vi "MS SQL_Read_STN_Count.vi"(8 "error in (no error)":errorcluster, 9 "Table?":string, 10 "Query":string, 11 "Refnum in":T1) -> (0 "error out":errorcluster, 1 "RFID":string[](array[string]), 2 "Count":i64, 3 "Refnum out":T1)   [LabVIEW 2020]
uses:
  <vilib>/addons/database/Connection.llb/Conn ObjectReference.ctl
  <vilib>/addons/database/NI_Database_API.lvlib
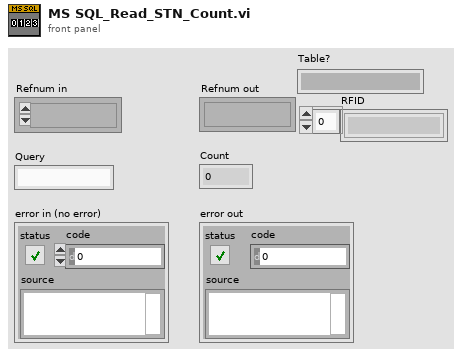
[diagram p1: front panel]
types:
  T1 = typedef "NI_Database_API.lvlib/Conn ObjectReference.ctl" = refnum<k1>
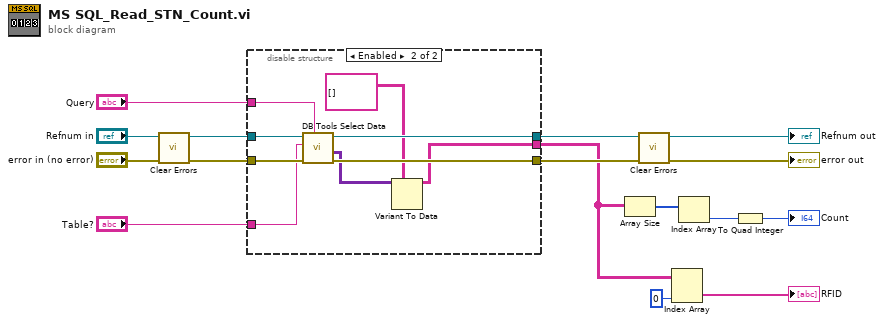
[diagram p0: block diagram]
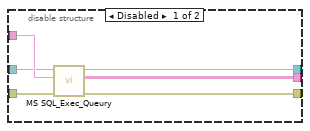
[diagram p2: hidden frame]
diagram:
  n1 = call <vilib>:"Clear Errors.vi"("error in (no error)"="error in (no error)") -> ("error out"=w1:errorcluster)  [unwired: 5 in, 1 out]
  n2 = disable-structure shown="Enabled" {
    disable-tunnel: [w20 w22] -> w4
    disable-tunnel: "Query" -> [w19 w28]
    disable-tunnel: "Refnum in" -> [w18 w29]
    disable-tunnel: w1 -> [w17 w27]
    disable-tunnel: [w16 w26] -> w11
    disable-tunnel: [w15 w25] -> w10
    disable-tunnel: "Table?" -> [_ w21]
    frame Disabled {
      n3 = call "MS SQL_Exec_Queury.vi"("error in (no error)"=w17, "Query"=w19, "Refnum in"=w18) -> ("error out"=w15:errorcluster, "Data"=w20:string[][], "Refnum out"=w16:T1)  [unwired: 5 in, 1 out]
    }
    frame Enabled {
      n4 = call <vilib>:"DB Tools Select Data.vi"("condition"=w28, "error in (no error)"=w27, "table"=w21, "connection reference"=w29) -> ("error out"=w25:errorcluster, "data"=w24:variant[][], "connection reference out"=w26:T1)  [unwired: 2 in]
      n5 = Variant To Data(type=string[][] [] ("Data"), Variant=w24) -> (data=w22:string[][])  [unwired: 1 in, 1 out]
    }
  }
  "Refnum out" <- w11
  n6 = Array Size(array=w4) -> (size(s)=w8:i32[])
  n7 = call <vilib>:"Clear Errors.vi"("error in (no error)"=w10) -> ("error out"=→"error out":errorcluster)  [unwired: 5 in, 1 out]
  n8 = Index Array(array=w4, index (col)=0 ("disabled index (col)")) -> (element=→"RFID":string[])  [unwired: 1 in]
  n9 = Index Array(array=w8) -> (element=w7:i32)  [unwired: 1 in]
  n10 = To Quad Integer(1:w7) -> (0:→"Count":i64)
